vi "rs3 is advanced mode enabled.vi"(8 "error in (no error)":errorcluster, 11 "device in":u64) -> (0 "error out":errorcluster, 1 "error":u64, 2 "enable?":i32, 3 "device out":u64)   [LabVIEW 2017, in "libRealSense3.lvlib"]
doc: "Queries whether the device is in ADVANCED MODE. If it is not, then it will not be possible to set many of the advanced depth and color settings. \n\nINPUT: \nDev in Input device\n\nOUTPUT:\nEnable? Is it enabled\nerror Error=0 is no error"
uses:
  <vilib>/addons/RealSense/libRealSense3.lvlib
  Users/Greg McKaskle/Downloads/librealsense-1.12.1/librealsense-1.12.1/bin/Win32/realsense-d.dll
panel:
  # "RS3 is Advanced Mode Enabled"
  # "(C) 2017 Intel Corp.,  AGJ"
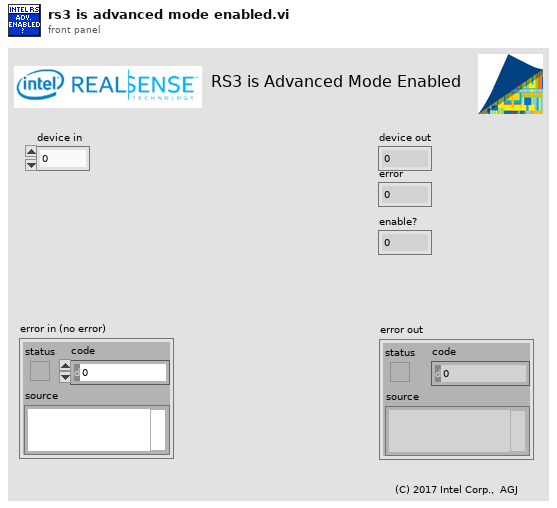
[diagram p1: front panel]
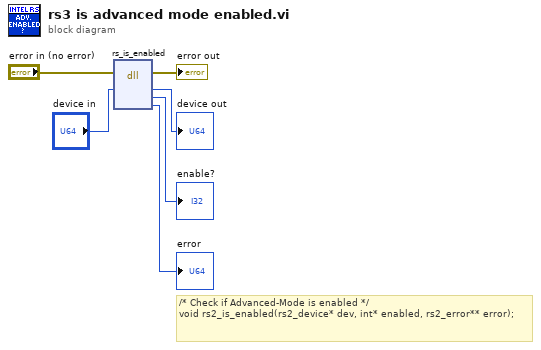
[diagram p0: block diagram]
diagram:
  # "/* Check if Advanced-Mode is enabled */\nvoid rs2_is_enabled(rs2_device* dev, int* enabled, rs2_error** error);"
  n1 = dll-call lib="C:/Users/Greg McKaskle/Downloads/librealsense-1.12.1/librealsense-1.12.1/bin/Win32/realsense-d.dll" fn="rs_is_enabled"(error in="error in (no error)", "device in"="device in") -> (error out=→"error out":errorcluster, "device in"=→"device out":u64, "enable?"=→"enable?":i32, "error"=→"error":u64)  [unwired: 5 in, 1 out]
